vi "pathplan.vi"() -> ()   [LabVIEW 2016]
panel:
  out "起点监视3":sgl[](array[numeric])
  in  "目标位置3":dbl[](array[numeric])=[2645.0, 2645.0]
  out "Key1（移动5）":bool
  in  "全场定位串口":refnum<visa-resource-name>="ASRL4::INSTR" caption="全场定位模块"
  in  "speed_max":dbl=15000.0
  in  "发送写入":refnum<visa-resource-name>
  in  "车宽的一半":dbl=200.0
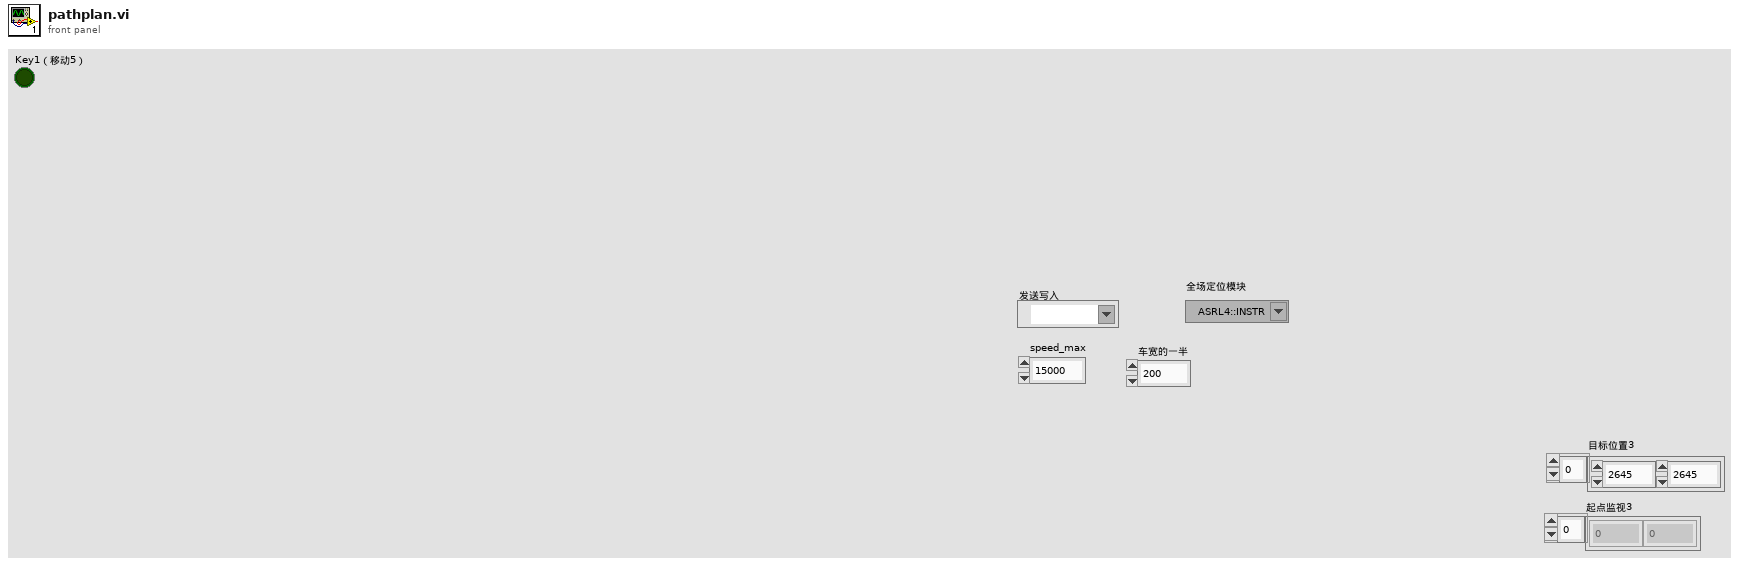
[diagram p1: front panel]
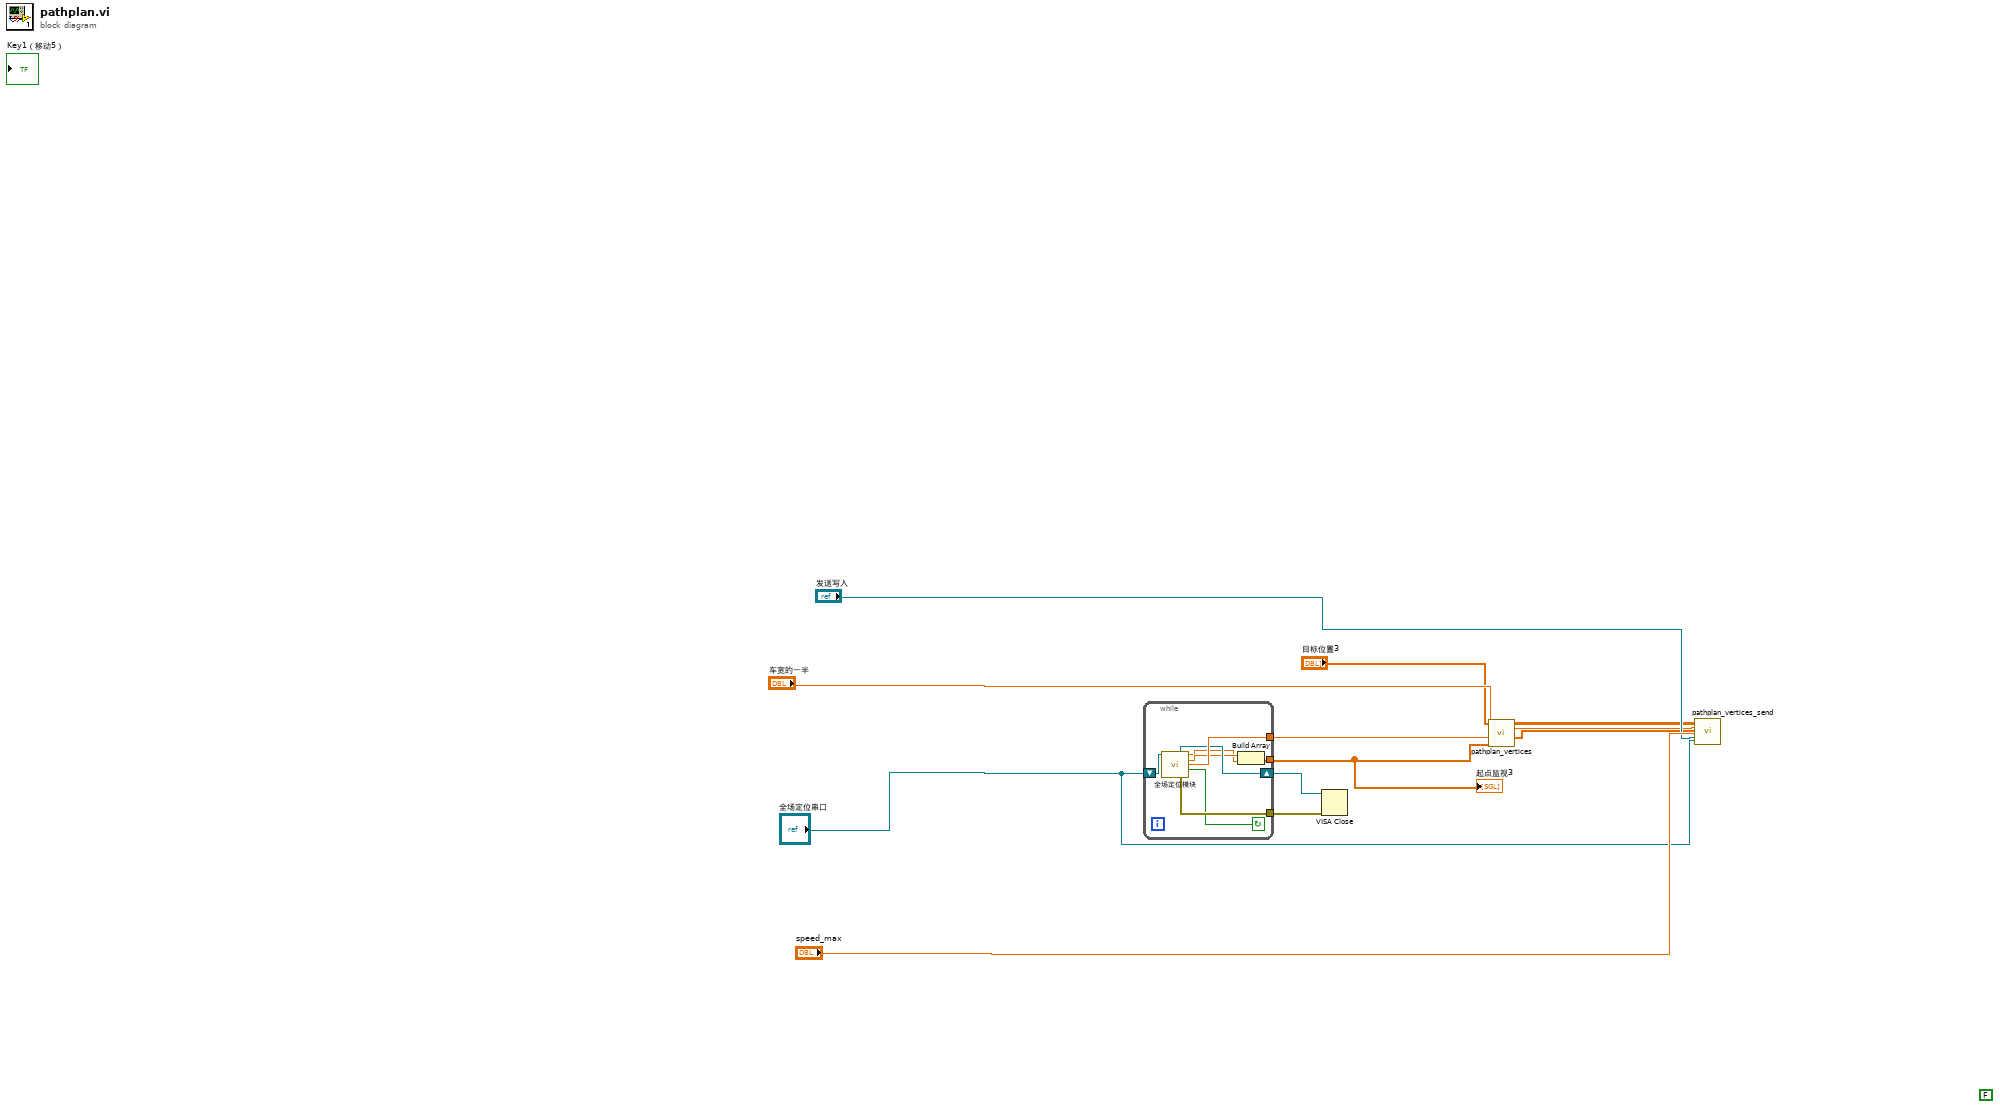
[diagram p0: block diagram]
diagram:
  (unwired) FALSE
  n1 = while {
    tunnel: [w20] -> w8
    tunnel: [w18] -> w6
    tunnel: [w17] -> w5
    shift-right: [w16] -> w4
    shift-left: "全场定位串口" -> [w19]
    stop <- w15 continue-if-true
    n2 = call "全场定位模块.vi"("VISA resource name"=w19) -> ("VISA资源名称输出"=w16:refnum<visa-resource-name>, "y"=w13:sgl, "x"=w14:sgl, "Zangle"=w17:sgl, "pd"=w15:bool, "错误输出2"=w18:errorcluster)  [unwired: 8 in, 1 out]
    n3 = Build Array(w14, w13) -> (w20:sgl[])
  }
  "起点监视3" <- w8
  n4 = VISA Close(VISA resource name=w4, error in (no error)=w6) -> ()  [unwired: 1 out]
  n5 = call "pathplan_vertices.vi"("终点"="目标位置3", "车宽的一半"="车宽的一半", "z_angle"=w5, "起点"=w8) -> ("vertices"=w3:dbl[][], "distance_all"=w2:dbl, "angle_all"=w1:dbl[])  [unwired: 3 in, 1 out]
  n6 = call "pathplan_vertices_send.vi"("vertices"=w3, "distance_all"=w2, "angle_all"=w1, "speed_max"="speed_max", "写入串口"="发送写入", "全场定位"="全场定位串口") -> ()  [unwired: 21 in, 1 out]
